vi "Select Waveform By Name.vi"(9 "NI_ChannelName":string, 11 "Array Of Wfm":waveform(dbl)[](array[waveform])) -> (1 "Found?":bool, 3 "Selected Wfm":waveform(dbl))   [LabVIEW 2024]
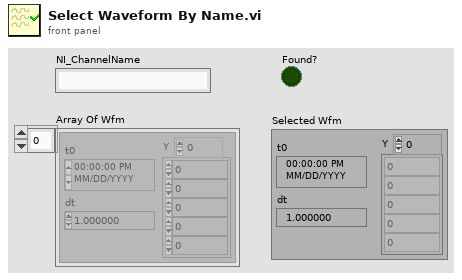
[diagram p1: front panel]
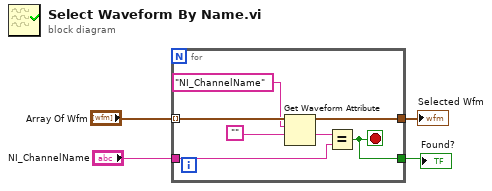
[diagram p0: block diagram]
diagram:
  n1 = for {
    tunnel: "Array Of Wfm" -> [w11] mode=indexing
    tunnel: "NI_ChannelName" -> [w7]
    tunnel: [w6] -> w2
    tunnel: [w5] -> w1
    stop <- w5 stop-if-true
    n2 = Get Waveform Attribute(5:"", 6:"NI_ChannelName" ("name"), 7:w11) -> (1:w8:string, 3:w6:waveform(dbl))  [unwired: 1 in, 2 out]
    n3 = Equal?(x=w8, y=w7) -> (x = y?=w5:bool)
  }
  "Selected Wfm" <- w2
  "Found?" <- w1
